vi "Normalizer_2_betas.vi"(0 "Acc":u64[][](array[numeric]), 3 "Time":dbl[](array[numeric]), 5 "Tamaño Sn":i32[](array[numeric]), 7 "AvgA":dbl, 11 "AvgB":dbl) -> (13 "bA_B":dbl, 14 "g(k)_2":dbl[][](array[numeric]), 16 "s(k)_n":dbl[][](array[numeric]), 18 "s(k)":dbl[][](array[numeric]), 19 "g(k)":dbl[][](array[numeric]))   [LabVIEW 2015]
uses:
  <vilib>/Analysis/Matrix/Numeric/Conversions/Matrix To Array - RM.vi
  <vilib>/Analysis/Matrix/NI_Matrix.lvlib
  <vilib>/Analysis/NI_AALPro.lvlib
panel:
  out "x/y":dbl[][](array[numeric])
  out "primeros elementos":dbl[](array[numeric])
  out "bA_B":dbl
  out "offset 2":dbl
  out "element":i32
  out "size(s)":i32[](array[numeric])
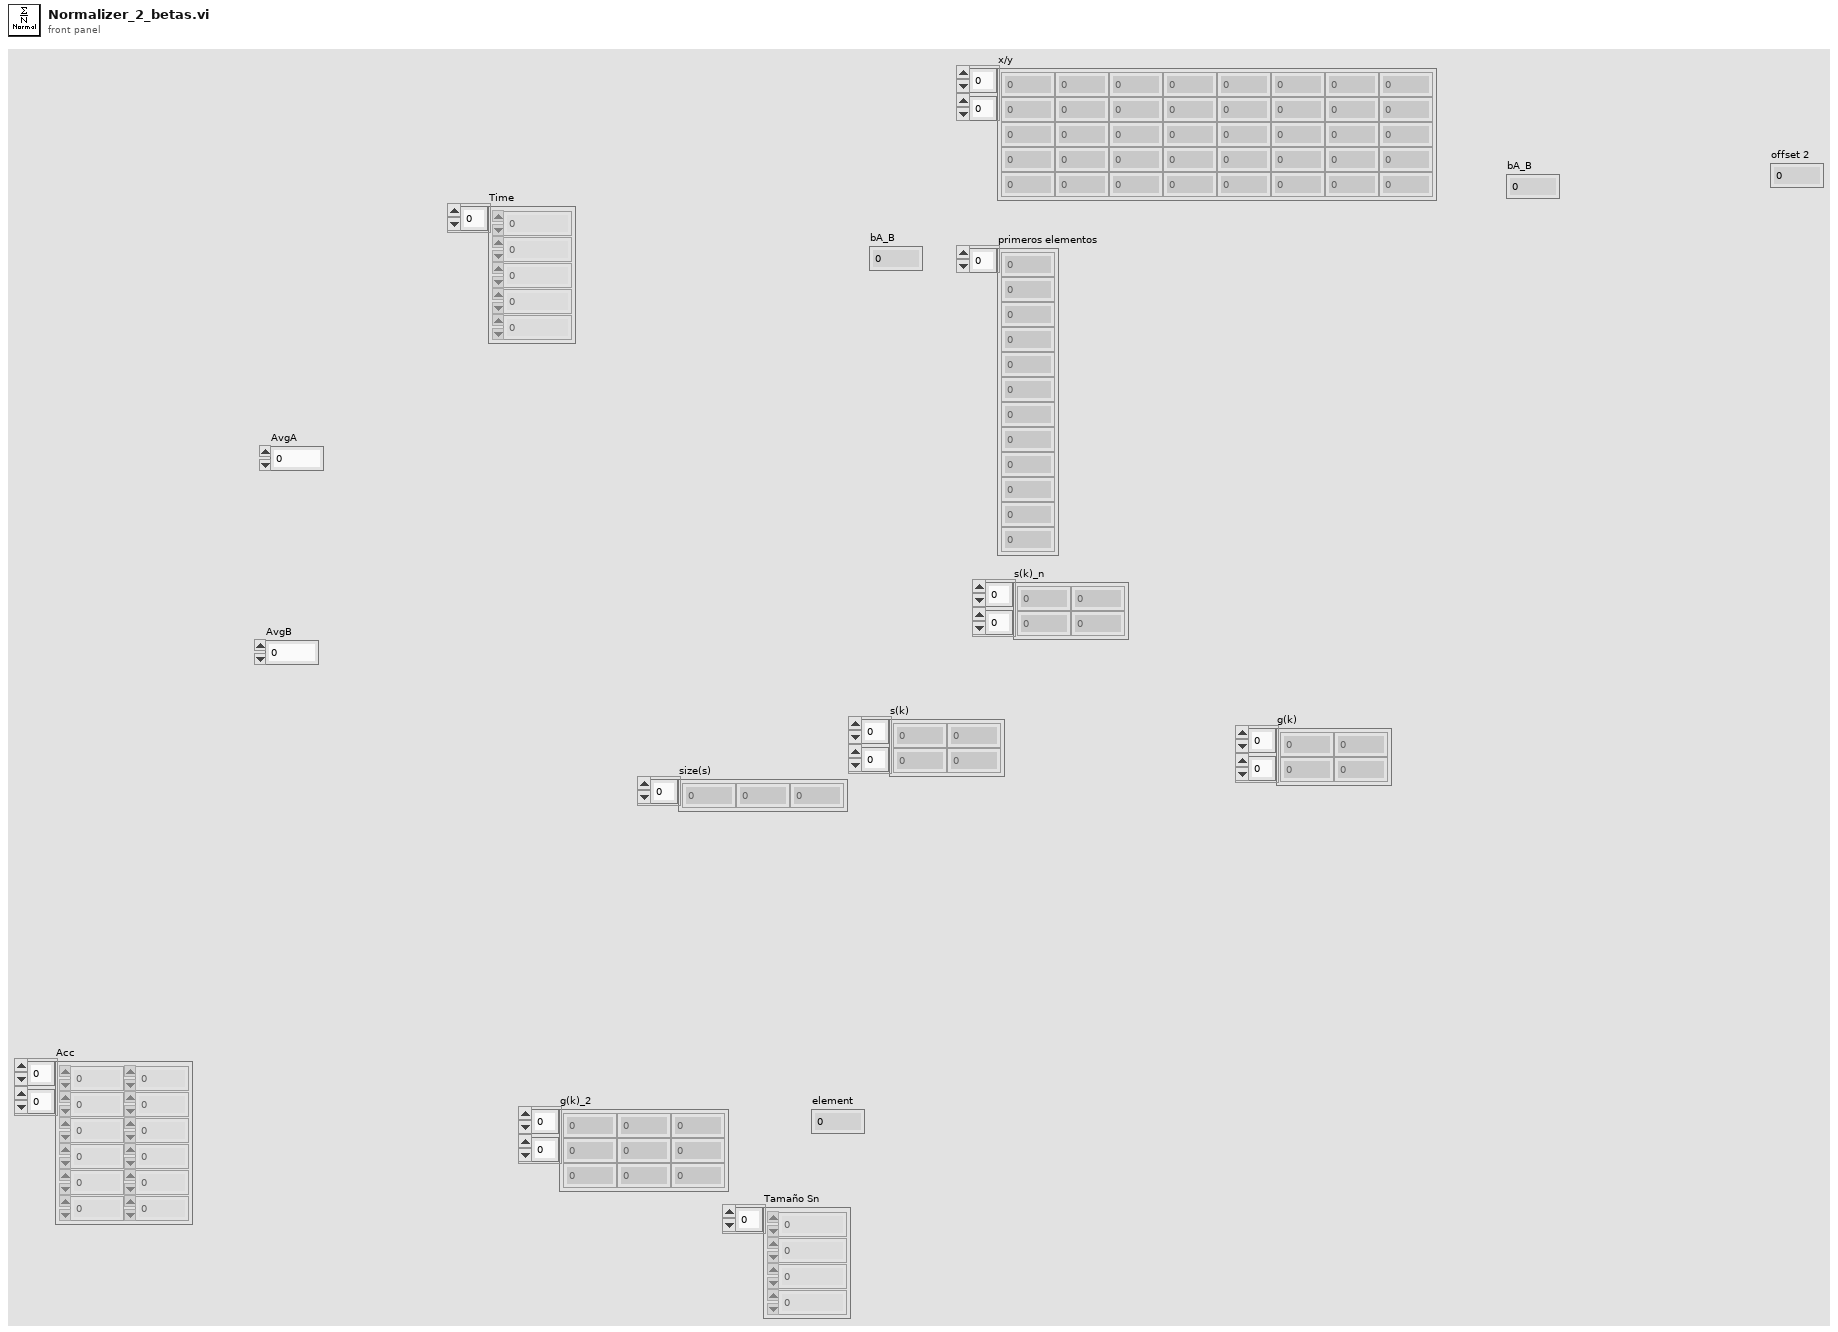
[diagram p1: front panel]
types:
  T1 = typedef "NI_Matrix.lvlib/RealMatrix.ctl" = dbl[][]
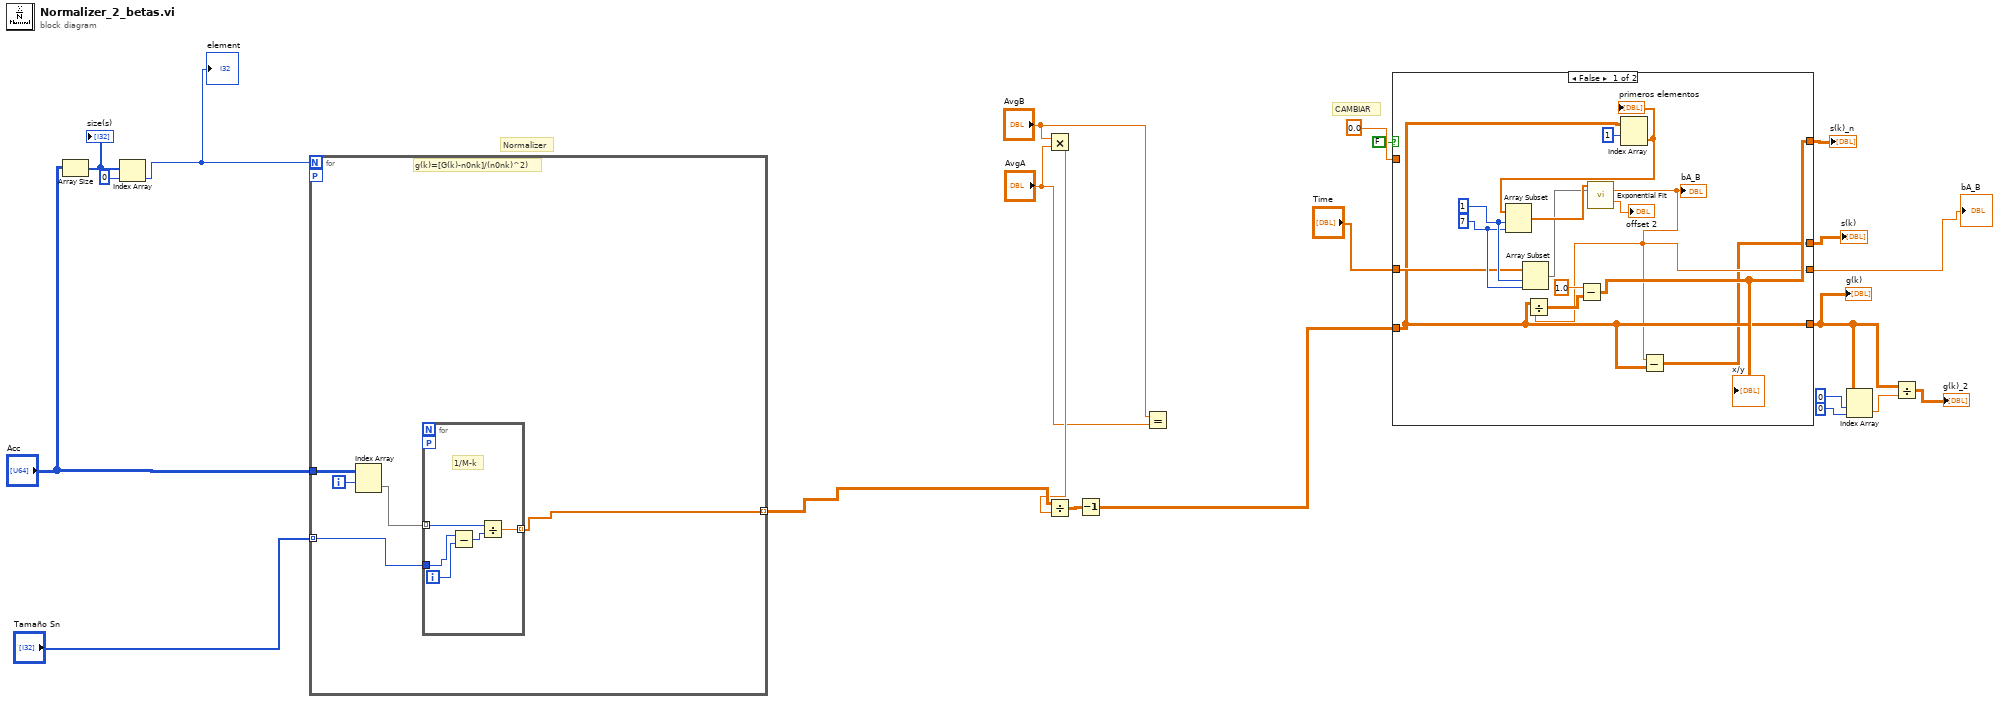
[diagram p0: block diagram]
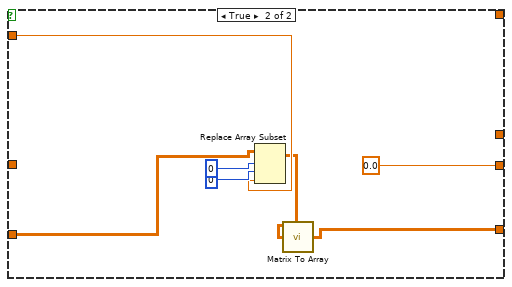
[diagram p2: hidden frame]
diagram:
  # "CAMBIAR"
  # "Normalizer"
  n1 = Array Size(array="Acc") -> (size(s)=w21:i32[])
  "size(s)" <- w21
  n2 = Index Array(array=w21, index=0) -> (element=w16:i32)
  "element" <- w16
  n3 = for {
    N: w16 -> [_]
    tunnel: "Acc" -> [w25]
    tunnel: "Tamaño Sn" -> [w27] mode=indexing
    tunnel: [w23] -> w18 mode=indexing
    workers-P: _ -> [_]
    i -> [w24]
    # "g(k)=[G(k)-n0nk]/(n0nk)^2)"
    n4 = Index Array(array=w25, index (row)=w24) -> (element=w26:u64[])  [unwired: 1 in]
    n5 = for {
      tunnel: [w32] -> w23 mode=indexing
      tunnel: w26 -> [w31] mode=indexing
      tunnel: w27 -> [w29]
      workers-P: _ -> [_]
      i -> [w28]
      # "1/M-k"
      n6 = Subtract(x=w29, y=w28) -> (x-y=w30:i32)
      n7 = Divide(x=w31, y=w30) -> (x/y=w32:dbl)
    }
  }
  n8 = Multiply(x="AvgB", y="AvgA") -> (x*y=w14:dbl)
  n9 = Divide(x=w18, y=w14) -> (x/y=w20:dbl[][])
  n10 = Decrement(x=w20) -> (x-1=w4:dbl[][])
  n11 = Equal?(x="AvgB", y="AvgA") -> ()  [unwired: 1 out]
  n12 = case shown="False" FALSE {
    tunnel: [w36 _] -> w15
    tunnel: 0.0 ("bA") -> [_ w50]
    tunnel: w4 -> [w35 w53]
    tunnel: [w35 w48] -> w11
    tunnel: [w33 _] -> w5
    tunnel: [w34 0.0] -> w7
    tunnel: "Time" -> [w39 _]
    frame False {
      w45 = 7 ("length")
      w46 = 1 ("index")
      n13 = Array Subset(array=w39, index=w46, length=w45) -> (w42:dbl[])
      n14 = Index Array(array=w35, index (row)=1) -> (element=w40:dbl[])  [unwired: 1 in]
      "primeros elementos" <- w40
      n15 = Array Subset(array=w40, index=w46, length=w45) -> (w43:dbl[])
      n16 = call <vilib>:"Exponential Fit.vi"("Y"=w43, "X"=w42) -> ("amplitude"=w34:dbl, "offset"=→"offset 2":dbl)  [unwired: 8 in, 4 out]
      "bA_B" <- w34
      n17 = Divide(x=w35, y=w34) -> (x/y=w37:dbl[][])
      n18 = Subtract(x=1.0, y=w37) -> (x-y=w36:dbl[][])
      "x/y" <- w36
      n19 = Subtract(x=w34, y=w35) -> (x-y=w33:dbl[][])
    }
    frame True {
      n20 = Replace Array Subset(array=w53, new element=w50, index (row)=0, index (col)=0 ("disabled index (col)")) -> (w49:T1)
      n21 = call-poly <vilib>:"Matrix To Array.vi"("Real Matrix"=w49) -> ("Real 2D Array"=w48:dbl[][])
    }
  }
  "s(k)" <- w5
  "s(k)_n" <- w15
  "g(k)" <- w11
  "bA_B" <- w7
  n22 = Index Array(array=w11, index (row)=0, index (col)=0) -> (element=w8:dbl)
  n23 = Divide(x=w11, y=w8) -> (x/y=→"g(k)_2":dbl[][])
